vi "Read.Data.vi"(8 "error in (no error)":errorcluster, 11 "FpgaRunner in":refnum<class "FpgaRunner.lvclass">) -> (0 "error out":errorcluster, 2 "Array":u64[](array[numeric]), 3 "FpgaRunner out":refnum<class "FpgaRunner.lvclass">)   [LabVIEW 2020, in "FpgaRunner.lvclass"]
uses:
  FpgaRunner.lvclass
  FpgaRunner.lvclass/FpgaRunner.ctl
  <vilib>/Utility/error.llb/Error Cluster From Error Code.vi
  <vilib>/rvi/errors/niLvFpgaAdjustHostInterfaceError.vi
  <vilib>/rvi/interface/nirviMethod/nirviMethod.xnode
  <vilib>/FPGAPlugInAG/Dynamic/niLvFpga_ReadFifo_Dynamic.vi
  <vilib>/rvi/errors/niLvFpgaMergeErrorWithErrorCode.vi
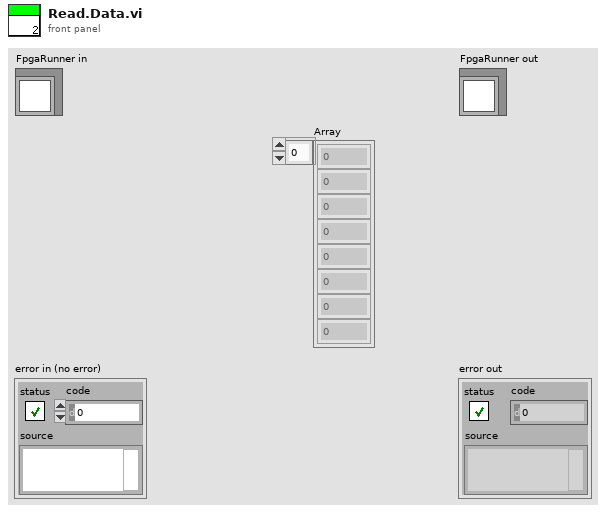
[diagram p1: front panel]
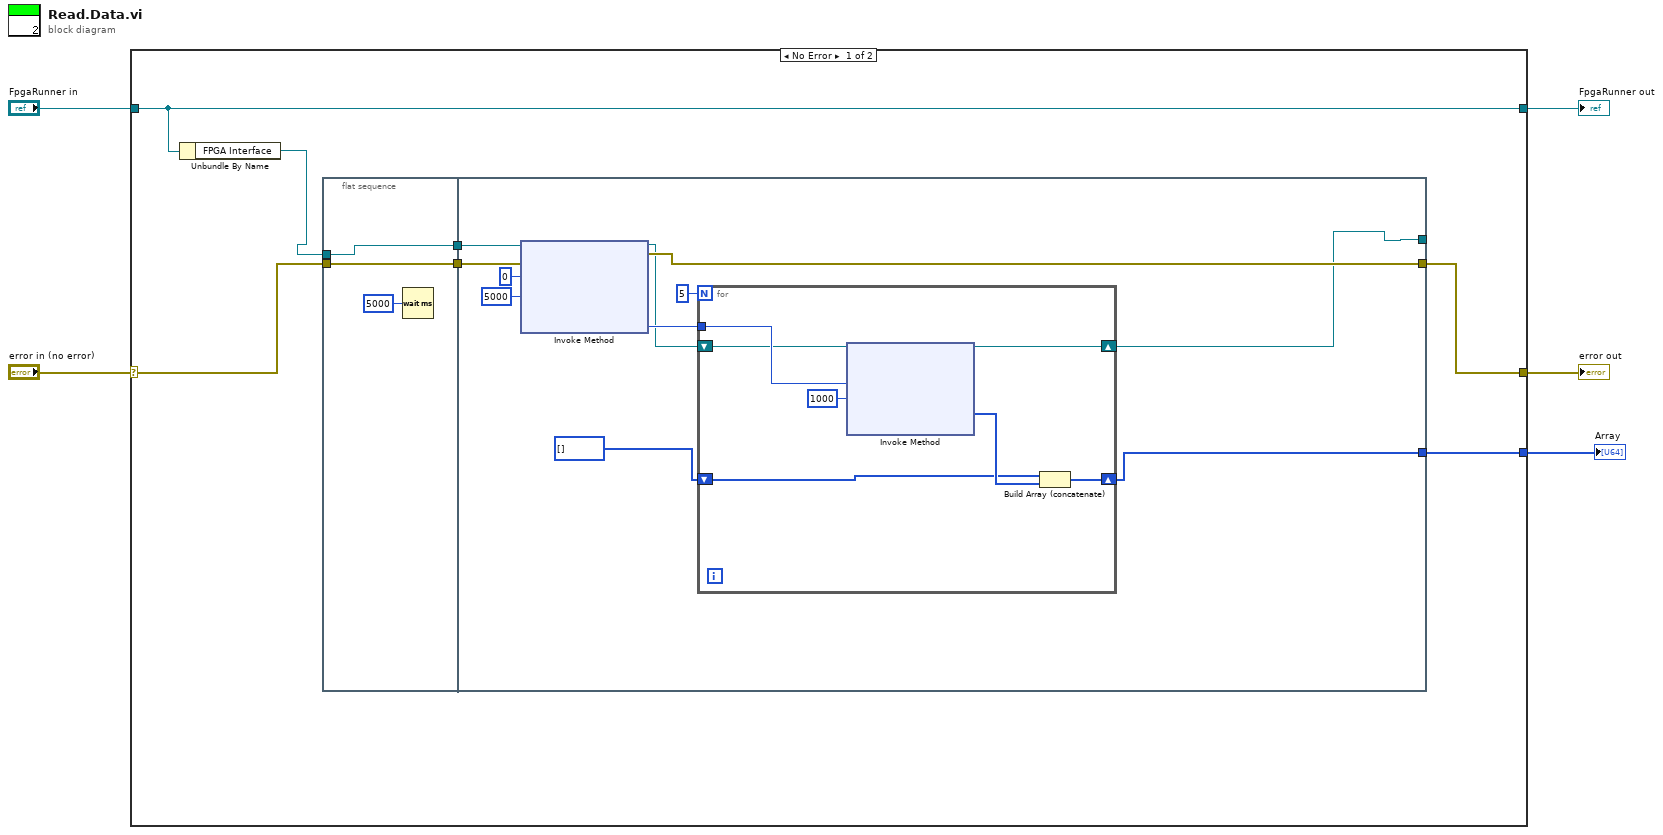
[diagram p0: block diagram]
diagram:
  n1 = case shown="No Error" "error in (no error)" {
    selector: "error in (no error)" -> [w10 w35]
    tunnel: [w9 w35] -> w4
    tunnel: [w8 w34] -> w2
    tunnel: "FpgaRunner in" -> [w8 w34]
    tunnel: [w6 _] -> w1
    frame No Error {
      n2 = Unbundle By Name(w8) -> ("FPGA Interface"=w7:refnum<k20>)
      n3 = flat-sequence {
        tunnel: [w14] -> w12
        tunnel: w10 -> [w14]
        tunnel: [w13] -> w11
        tunnel: w7 -> [w13]
        tunnel: w12 -> [w26]
        tunnel: w11 -> [w25]
        tunnel: [w24] -> w9
        tunnel: [w17] -> _
        tunnel: [w16] -> w6
        frame #0 {
          n4 = Wait (ms)(milliseconds to wait=u32 5000) -> ()  [unwired: 1 out]
        }
        frame #1 {
          n5 = xnode "Invoke Method"("FPGA VI Reference In"=w25, "error in"=w26, "Number of Elements"=u32 0, "Timeout (ms)"=5000) -> ("FPGA VI Reference Out"=w18:refnum<k20>, "error out"=w24:errorcluster, "Elements Remaining"=w20:u32)  [unwired: 1 out]
          n6 = for {
            N: 5 -> [_]
            tunnel: w20 -> [w33]
            shift-right: [w29] -> w16
            shift-left: u64[] [] -> [w30]
            shift-right: [w27] -> w17
            shift-left: w18 -> [w28]
            n7 = xnode "Invoke Method"("FPGA VI Reference In"=w28, "Number of Elements"=w33, "Timeout (ms)"=1000) -> ("FPGA VI Reference Out"=w27:refnum<k20>, "Data"=w31:u64[])  [unwired: 1 in, 2 out]
            n8 = Build Array (concatenate)(w30, w31) -> (w29:u64[])
          }
        }
      }
    }
    frame Error {
    }
  }
  "error out" <- w4
  "FpgaRunner out" <- w2
  "Array" <- w1
